vi "Error Handling - Process Error.vi"(9 "Exit on Error":bool, 10 "Ignore Errors":i32[](array[numeric]), 11 "error to process":errorcluster) -> (3 "Error Processed":bool)   [LabVIEW 2023, in "HAF.lvlib"]
doc: "Processes the error passed in. If on the ignore list, then nothing happens otherwise it places a message on the Notification Queue so that an appropriate action can be taken. If an error was passed in and not ignored then the Error flag is set for output otherwise it is flagged as no error."
uses:
  HAF.lvlib
  All Notification Message Ids.ctl
  Global Resources.vi
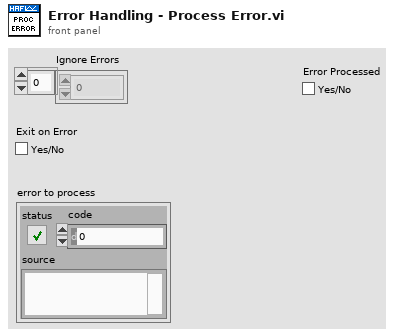
[diagram p1: front panel]
types:
  T1 = typedef "HAF.lvlib/All Message Queues.ctl" = cluster{"Internal":refnum<queue>, "Notifications":refnum<queue>}
  T2 = typedef "HAF.lvlib/All Notification Message Ids.ctl" = cluster{"Initialise":string, "Exit":string, "Error":string, "Result":string, "Done":string}
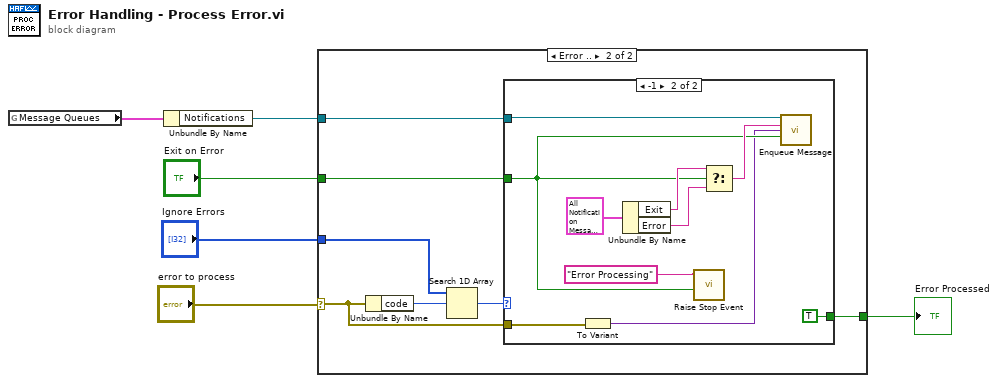
[diagram p0: block diagram]
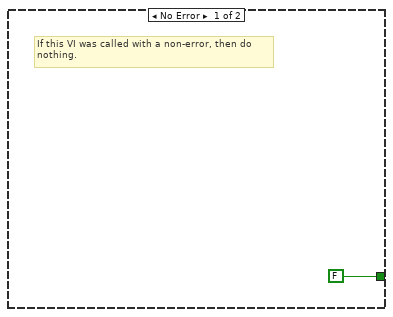
[diagram p2: hidden frame]
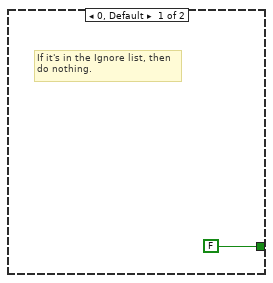
[diagram p3: hidden frame]
diagram:
  n1 = global read "Global Resources.vi" "Message Queues"() -> (w6:T1)
  n2 = Unbundle By Name(w6) -> ("Notifications"=w3:refnum<queue>)
  n3 = case shown="Error .." "error to process" {
    selector: "error to process" -> [_ w8]
    tunnel: [FALSE w11] -> w1
    tunnel: "Ignore Errors" -> [_ w13]
    tunnel: w3 -> [_ w10]
    tunnel: "Exit on Error" -> [_ w9]
    frame No Error {
      # "If this VI was called with a non-error, then do\nnothing."
    }
    frame Error {
      n4 = Unbundle By Name(w8) -> ("code"=w14:i32)
      n5 = Search 1D Array(1D array=w13, element=w14) -> (index of element=w12:i32)  [unwired: 1 in]
      n6 = case shown="-1" w12 {
        tunnel: [FALSE TRUE] -> w11
        tunnel: w10 -> [_ w22]
        tunnel: w9 -> [_ w19]
        tunnel: w8 -> [_ w18]
        frame 0, Default {
          # "If it's in the Ignore list, then\ndo nothing."
        }
        frame -1 {
          n7 = To Variant(anything=w18) -> (Variant=w17:variant)
          n8 = Unbundle By Name(T2 {"Initialise"="Initialise", "Exit"="Exit", "Error"="Error", "Result"="Result", "Done"="Done"} ("Message IDs")) -> ("Exit"=w24:string, "Error"=w23:string)
          n9 = call "Raise Stop Event.vi"("Send Stop"=w19, "Raiser Name"="Error Processing") -> ()  [unwired: 9 in, 1 out]
          n10 = Select(t=w24, s=w19, f=w23) -> (s? t:f=w21:string)
          n11 = call "Enqueue Message.vi"("Message Queue In"=w22, "Message Id"=w21, "Message Data"=w17, "Priority"=w19) -> ()  [unwired: 10 in, 2 out]
        }
      }
    }
  }
  "Error Processed" <- w1
